vi "DeleteALL.vi"(8 "error in (no error)":errorcluster) -> (0 "error out":errorcluster)   [LabVIEW 2020, in "Settings.lvlib"]
uses:
  Settings.lvlib
  <vilib>/drjdpowell/SQLite Library/SQL Connection/Open (path).vi
  <vilib>/drjdpowell/SQLite Library/SQL Connection/Open (string).vi
  <vilib>/AdvancedString/Path To Command Line String.vi
  <vilib>/drjdpowell/SQLite Library/SQL Connection/Execute SQL (No results).vi
  <vilib>/drjdpowell/SQLite Library/SQL Connection/Connection.lvclass
  <vilib>/drjdpowell/SQLite Library/SQLite.lvlib
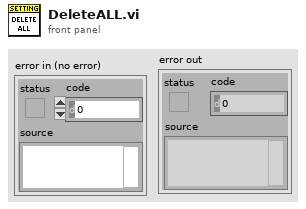
[diagram p1: front panel]
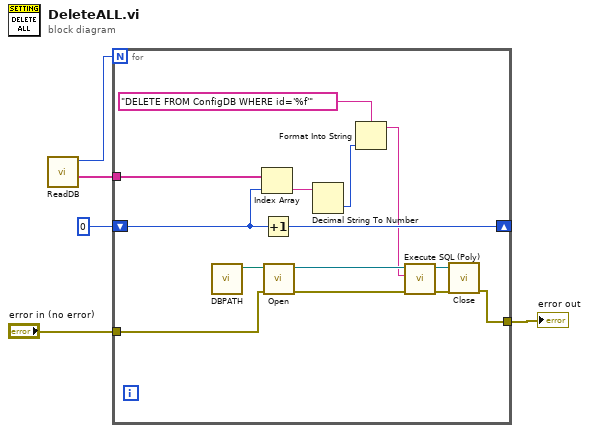
[diagram p0: block diagram]
diagram:
  n1 = call "ReadDB.vi"() -> ("IDS"=w3:string[], "Max ID"=w5:i32)  [unwired: 8 in, 2 out]
  n2 = for {
    N: w5 -> [_]
    shift-right: [w19] -> _
    shift-left: 0 -> [w18]
    tunnel: w3 -> [w17]
    tunnel: [w9] -> w2
    tunnel: "error in (no error)" -> [w8]
    n3 = call "DBPATH.vi"() -> ("appended path"=w14:path)  [unwired: 11 in]
    n4 = Index Array(array=w17, index=w18) -> (element=w15:string)
    n5 = Increment(x=w18) -> (x+1=w19:i32)
    n6 = call-poly <vilib>:"Open.vi"("error in (no error)"=w8, "db file"=w14) -> ("error out"=w10:errorcluster, "SQLite Connection"=w12:refnum<class "Connection.lvclass">)  [unwired: 8 in]
    n7 = Decimal String To Number(string=w15) -> (number=w6:i32)  [unwired: 2 in, 1 out]
    n8 = Format Into String(format string="DELETE FROM ConfigDB WHERE id='%f'" ("SQL"), w6) -> (resulting string=w7:string)  [unwired: 2 in, 1 out]
    n9 = call-poly <vilib>:"Execute SQL (Poly).vi"("error in (no error)"=w10, "SQL"=w7, "SQLite Connection in"=w12) -> ("error out"=w11:errorcluster, "SQLite Connection"=w13:refnum<class "Connection.lvclass">)  [unwired: 7 in]
    n10 = call-dynamic "Close.vi"("error in (no error)"=w11, "SQLite Connection in"=w13) -> ("error out"=w9:errorcluster)  [unwired: 9 in]
  }
  "error out" <- w2
